vi "Search.vi"(7 "Parent ID":string, 8 "Error In":errorcluster, 10 "Name or Tree Path":string, 11 "Tree Manager":T1) -> (0 "Error Out":errorcluster, 3 "Tree Manager":T1, 5 "IDs":string[](array[string]))   [LabVIEW 2020, in "NI_VIAnCFGDataStructure.lvlib" / "Tree.lvclass"]
doc: "Search through the Tree Manager to find a Tree with a specific name. \n\nIf the Parent ID is wired the search will be shallow, limited to only the Children of the Parent Tree and the Name or Tree Path input will expect a name.\n\nIf the Parent ID is <b>NOT</b> wired a global search will be performed, through all Trees, unless an optimization has been run before. If the Tree is optimized a look-up will be performed instead and the Name or Tree Path input can be provided as either. The Tree Path has to begin at a Root Tree.\n\nThe returned array of IDs contains the IDs of <b>ALL</b> Trees with a matching name."
uses:
  <vilib>/addons/analyzer/VIAnCFGDataStructure/Tree Manager/Tree.lvclass
  <vilib>/addons/analyzer/VIAnCFGDataStructure/Tree Manager/Typedefs/Session Handle.ctl
  <vilib>/addons/analyzer/VIAnCFGDataStructure/Tree Manager/Tree.lvclass/Tree.ctl
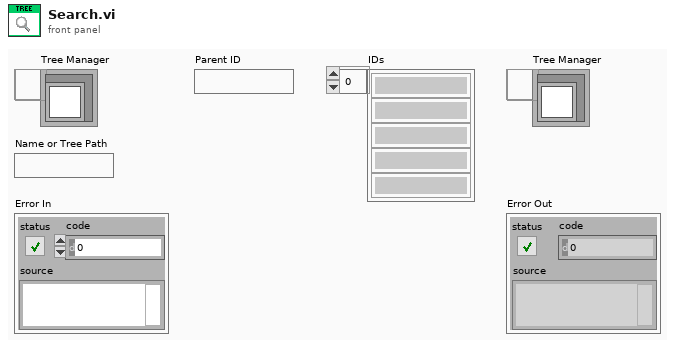
[diagram p1: front panel]
types:
  T1 = typedef "NI_VIAnCFGDataStructure.lvlib/Tree.lvclass/Session Handle.ctl" = refnum<data-value>
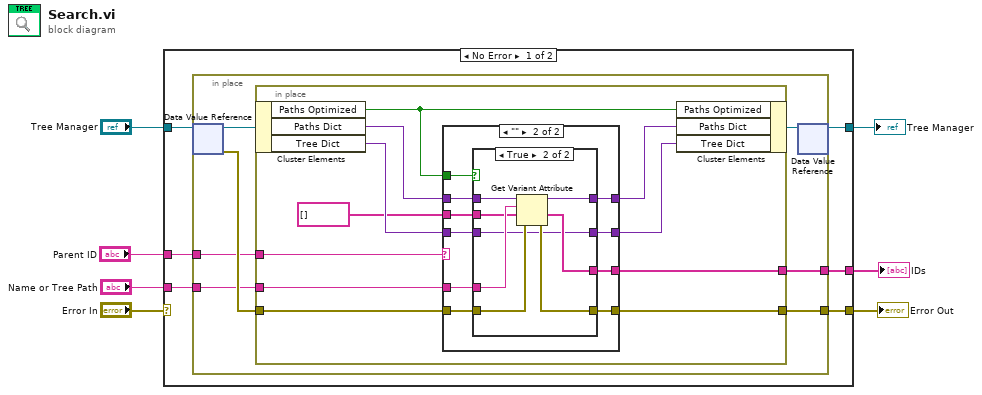
[diagram p0: block diagram]
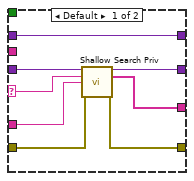
[diagram p2: hidden frame]
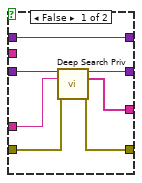
[diagram p3: hidden frame]
diagram:
  n1 = case shown="No Error" "Error In" {
    selector: "Error In" -> [_ w65]
    tunnel: "Tree Manager" -> [w13 w66]
    tunnel: [w12 w66] -> w6
    tunnel: [w11 w65] -> w4
    tunnel: "Parent ID" -> [w10 _]
    tunnel: "Name or Tree Path" -> [w9 _]
    tunnel: [w8 _] -> w1
    frame No Error {
      n2 = in-place {
        in-place-border: [w20] -> w11
        in-place-border: w10 -> [w18]
        in-place-border: w9 -> [w17]
        in-place-border: [w16] -> w8
        n3 = in-place-dvr #1(w13) -> (w15:refnum<class "Tree.lvclass">, w19:errorcluster)
        n4 = in-place {
          in-place-border: [w31] -> w20
          in-place-border: w19 -> [w30]
          in-place-border: w18 -> [w23]
          in-place-border: w17 -> [w29]
          in-place-border: [w28] -> w16
          n5 = in-place-cluster #2(w15) -> ("Paths Optimized"=w22:bool, "Paths Dict"=w26:variant, "Tree Dict"=w24:variant)
          n6 = case shown="\"\"" w23 {
            selector: w23 -> [w39 _]
            tunnel: w24 -> [w38 w48]
            tunnel: [w37 w43] -> w25
            tunnel: w30 -> [w33 w46]
            tunnel: [w35 w45] -> w31
            tunnel: w29 -> [w34 w47]
            tunnel: [w36 w44] -> w28
            tunnel: w26 -> [w32 w41]
            tunnel: [w32 w42] -> w27
            tunnel: w22 -> [_ w49]
            tunnel: string[] [] ("IDs") -> [_ w40]
            frame Default {
              n7 = call <vilib>:"Shallow Search Priv.vi"("Tree Dictionary In"=w38, "Unique ID"=w39, "Name"=w34, "error in"=w33) -> ("Tree Dictionary Out"=w37:variant, "IDs"=w36:string[], "error out"=w35:errorcluster)  [unwired: 9 in]
            }
            frame "" {
              n8 = case shown="True" w49 {
                tunnel: w48 -> [w56 w58]
                tunnel: w47 -> [w55 w63]
                tunnel: w46 -> [w54 w62]
                tunnel: [w53 w61] -> w45
                tunnel: [w52 w60] -> w44
                tunnel: [w51 w58] -> w43
                tunnel: [w50 w59] -> w42
                tunnel: w41 -> [w50 w64]
                tunnel: w40 -> [_ w57]
                frame False {
                  n9 = call <vilib>:"Deep Search Priv.vi"("Tree Dictionary In"=w56, "Name"=w55, "error in"=w54) -> ("Tree Dictionary Out"=w51:variant, "IDs"=w52:string[], "error out"=w53:errorcluster)  [unwired: 10 in]
                }
                frame True {
                  n10 = Get Variant Attribute(Variant=w64, name=w63, default value (empty Variant)=w57, error in=w62) -> (duplicate Variant=w59:variant, value=w60:string[], error out=w61:errorcluster)  [unwired: 1 out]
                }
              }
            }
          }
          n11 = in-place-cluster #2("Paths Optimized"=w22, "Paths Dict"=w27, "Tree Dict"=w25) -> (w14:refnum<class "Tree.lvclass">)
        }
        n12 = in-place-dvr #1(w14) -> (w12:T1)  [unwired: 1 out]
      }
    }
    frame Error {
    }
  }
  "Tree Manager" <- w6
  "Error Out" <- w4
  "IDs" <- w1
